vi "GetTrafficLightRef.vi"(0 "object in":refnum<class "RedState.lvclass">, 5 "Error In":errorcluster) -> (14 "object out":refnum<class "RedState.lvclass">, 16 "TrafficLightRef":refnum<class "TrafficLight.lvclass">, 19 "Error Out":errorcluster)   [LabVIEW 2024, in "RedState.lvclass"]
uses:
  RedState.lvclass
  TrafficLight_class/TrafficLight.lvclass
  RedState.lvclass/RedState.ctl
panel:
  # "Connector Pane"
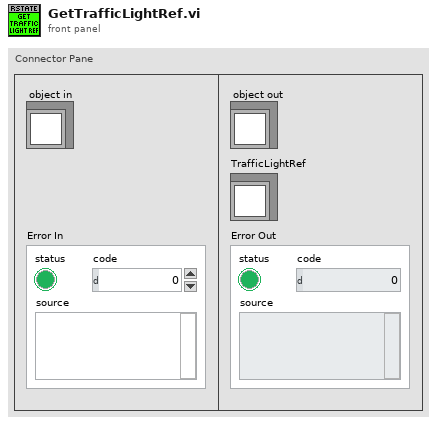
[diagram p1: front panel]
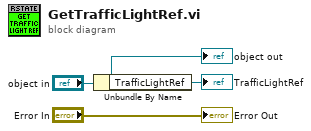
[diagram p0: block diagram]
diagram:
  n1 = Unbundle By Name("object in") -> ("TrafficLightRef"=→"TrafficLightRef":refnum<class "TrafficLight.lvclass">)
  "Error Out" <- "Error In"
  "object out" <- "object in"
